vi "E443X_ESG_VSG_ALC_Power_Search.vi"(0 "VISA Resource Name":refnum<visa-resource-name>, 1 "ALC BW (T:NORMAL)":bool=TRUE, 5 "ALC (T:ON)":bool=TRUE, 7 "Search Reference (0: Fixed)":u16(ring) items=["Fixed", "Modulated"], 9 "Power Search (F:MANUAL)":bool, 11 "error in (no error)":errorcluster {"code" format="%.0x"}) -> (4 "VISA Resource Name Out":refnum<visa-resource-name>, 15 "error out":errorcluster {"code" format="%.0x"})   [LabVIEW 2015]
doc: "This VI is used to turn the Automatic leveling control (ALC) on or off\nor to configure and start the Power Search internal calibration routine, used to achieve calibrated output power when the ALC is off.\n\nNote:\nYou do not need to disconnect modulation inputs, however modulation is disabled during powere search."
panel:
  # "NORMAL"
  # "NARROW"
  # "AUTO"
  # "MANUAL"
  # "ON"
  # "OFF"
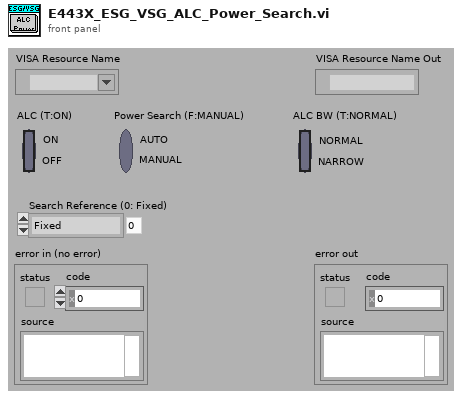
[diagram p1: front panel]
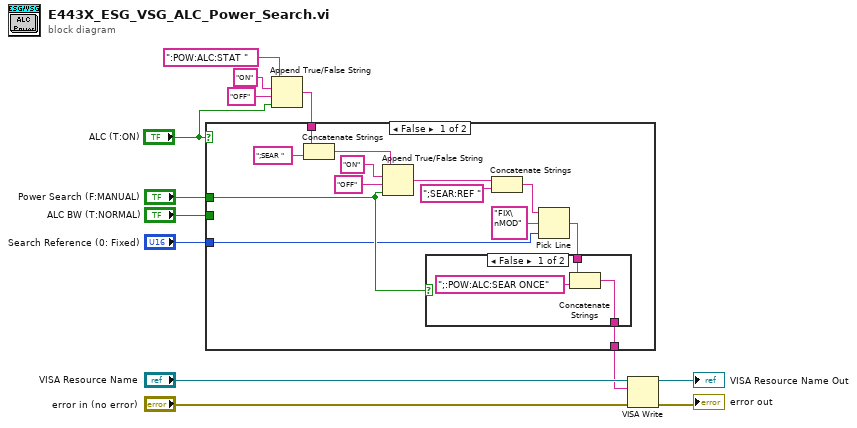
[diagram p0: block diagram]
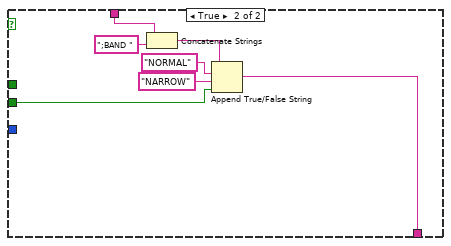
[diagram p3: hidden frame]
diagram:
  n1 = Append True/False String(1:"ALC (T:ON)", 2:"OFF" ("false string"), 3:"ON" ("true string"), 4:":POW:ALC:STAT ") -> (0:w6:string)
  n2 = case shown="False" "ALC (T:ON)" {
    tunnel: w6 -> [w22 w34]
    tunnel: "Power Search (F:MANUAL)" -> [w20 _]
    tunnel: [w21 w32] -> w2
    tunnel: "ALC BW (T:NORMAL)" -> [_ w31]
    tunnel: "Search Reference (0: Fixed)" -> [w18 _]
    frame False {
      n3 = Concatenate Strings(w22, ";SEAR ") -> (w25:string)
      n4 = Append True/False String(1:w20, 2:"OFF" ("false string"), 3:"ON" ("true string"), 4:w25) -> (0:w16:string)
      n5 = Concatenate Strings(w16, ";SEAR:REF ") -> (w14:string)
      n6 = Pick Line(string ("")=w14, multi-line string="FIX\nMOD", line index=w18) -> (output string=w17:string)
      n7 = case shown="False" w20 {
        tunnel: [w29 w30] -> w21
        tunnel: w17 -> [w27 w30]
        frame False {
          n8 = Concatenate Strings(w27, ";:POW:ALC:SEAR ONCE") -> (w29:string)
        }
        frame True {
        }
      }
    }
    frame True {
      n9 = Concatenate Strings(w34, ";BAND ") -> (w33:string)
      n10 = Append True/False String(1:w31, 2:"NARROW" ("false string"), 3:"NORMAL" ("true string"), 4:w33) -> (0:w32:string)
    }
  }
  n11 = VISA Write(VISA resource name="VISA Resource Name", write buffer=w2, error in (no error)="error in (no error)") -> (VISA resource name out=→"VISA Resource Name Out":refnum<visa-resource-name>, error out=→"error out":errorcluster)  [unwired: 1 out]
